vi "Single Video Display2.vi"() -> ()   [LabVIEW 2017]
uses:
  VideoWindowsCommand.ctl
panel:
  in  "Video Feed":enum16{"Camera 1", "Camera2", "Mobile"}(ring)=enum."Camera2"
  in  "MozillaBrowser 2":refnum<k7>(container)
  in  "Exit":bool
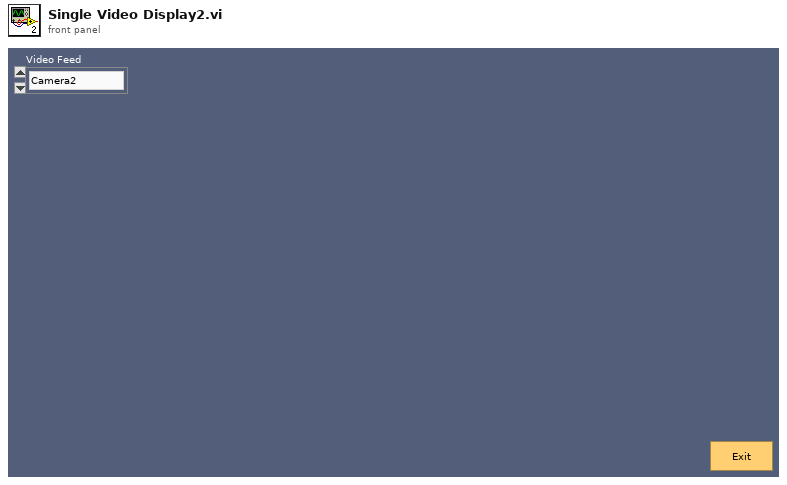
[diagram p1: front panel]
types:
  T1 = typedef "VideoWindowsCommand.ctl" = cluster{"Position":cluster{"Right":i32, "Bottom":i32}, "Exit":bool, "MoveToFront":bool}
  T2 = typedef "LVRectTypeDef.ctl" = cluster{"Left":i16, "Top":i16, "Right":i16, "Bottom":i16}
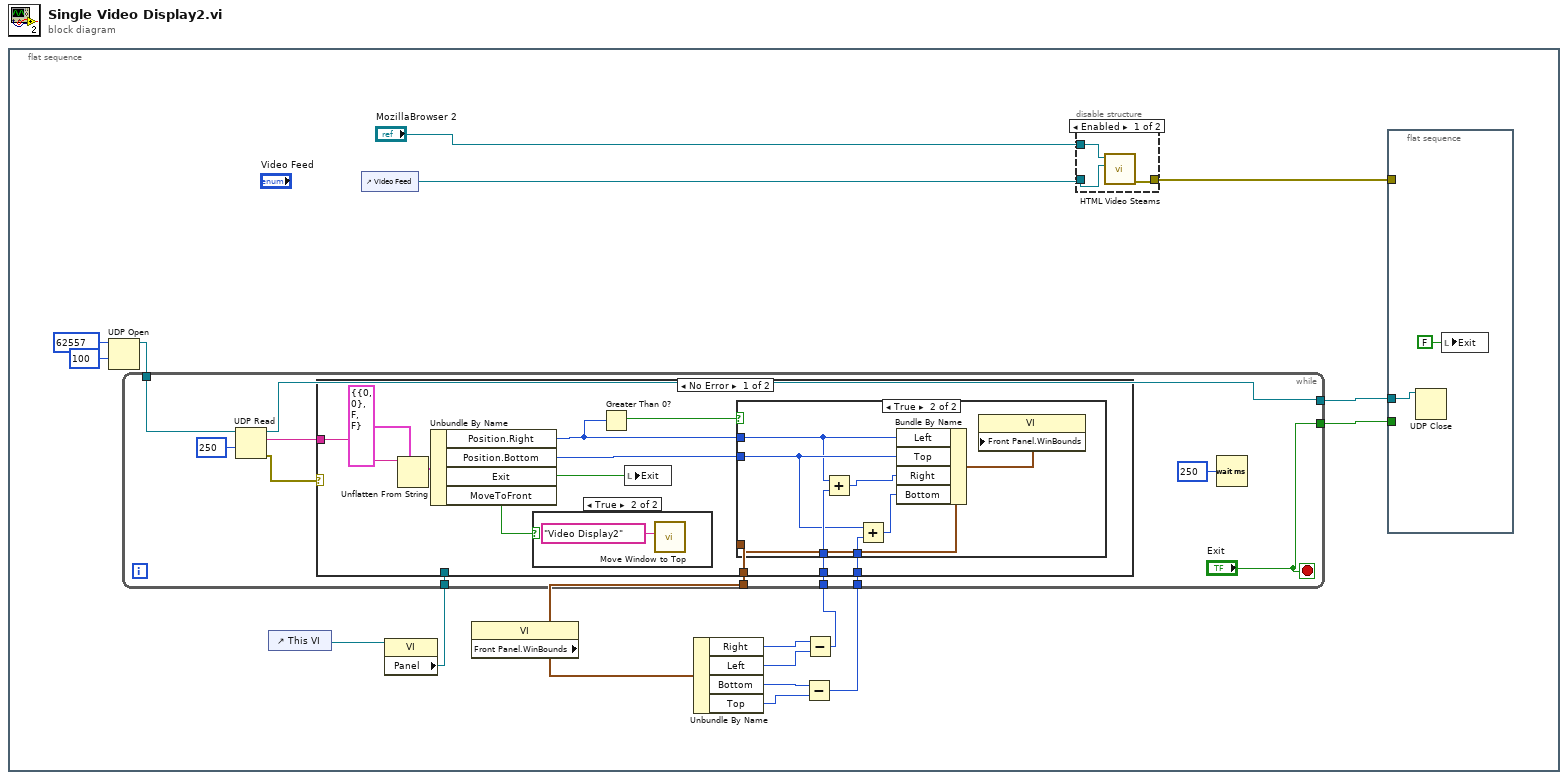
[diagram p0: block diagram]
diagram:
  n1 = flat-sequence {
    frame #0 {
      n2 = UDP Open(9:100 ("timeout ms (25000)"), 11:u16 62557 ("port")) -> (port=w12:refnum<k16>)  [unwired: 3 in, 2 out]
      n3 = control-ref of="This VI"() -> (w11:refnum<vi>)
      n4 = control-ref of="Video Feed"() -> (w16:refnum<vi>)
      n5 = property class="VI"(reference=w11) -> ("Panel"=w10:refnum<vi>)  [unwired: 1 in, 2 out]
      n6 = property class="VI"() -> ("Front Panel.WinBounds"=w3:T2)  [unwired: 2 in, 2 out]
      n7 = Unbundle By Name(w3) -> ("Right"=w6:i16, "Left"=w7:i16, "Bottom"=w4:i16, "Top"=w5:i16)
      n8 = Subtract(x=w4, y=w5) -> (x-y=w1:i16)
      n9 = Subtract(x=w6, y=w7) -> (x-y=w2:i16)
      n10 = while {
        tunnel: ["Exit"] -> w14
        tunnel: w12 -> [w28]
        tunnel: w10 -> [w24]
        tunnel: [w23] -> w9
        tunnel: w3 -> [w22]
        tunnel: w2 -> [w21]
        tunnel: w1 -> [w20]
        stop <- "Exit" stop-if-true
        n11 = UDP Read(connection ID=w28, timeout ms (25000)=250) -> (data out=w25:string, error out=w26:errorcluster, 3:w23:refnum<k16>)  [unwired: 2 in, 2 out]
        n12 = case shown="No Error" w26 {
          tunnel: w25 -> [w41 _]
          tunnel: w24 -> [_ _]
          tunnel: w22 -> [w37 _]
          tunnel: w21 -> [w36 _]
          tunnel: w20 -> [w34 _]
          frame No Error {
            n13 = Unflatten From String(type=T1 {"Position"={"Right"=0, "Bottom"=0}, "Exit"=FALSE, "MoveToFront"=FALSE}, binary string=w41) -> (value=w39:T1)  [unwired: 3 in, 2 out]
            n14 = Unbundle By Name(w39) -> ("Position.Right"=w33:i32, "Position.Bottom"=w35:i32, "Exit"=w38:bool, "MoveToFront"=w31:bool)
            n15 = case shown="True" w31 {
              frame False {
              }
              frame True {
                n16 = call "Move Window to Top.vi"("window name (\"\")"="Video Display2" ("window name (\"\")")) -> ()  [unwired: 5 in, 2 out]
              }
            }
            n17 = Greater Than 0?(x=w33) -> (x > 0?=w32:bool)
            n18 = local write "Exit"(w38) -> ()
            n19 = case shown="True" w32 {
              tunnel: w37 -> [_ w50]
              tunnel: w36 -> [_ w49]
              tunnel: w35 -> [_ w47]
              tunnel: w34 -> [_ w46]
              tunnel: w33 -> [_ w43]
              frame False {
              }
              frame True {
                n20 = Add(x=w43, y=w49) -> (x+y=w48:i32)
                n21 = Add(x=w47, y=w46) -> (x+y=w45:i32)
                n22 = Bundle By Name(cluster=w50, "Left"=w43, "Top"=w47, "Right"=w48, "Bottom"=w45) -> (w44:T2)
                n23 = property class="VI"("Front Panel.WinBounds"=w44) -> ()  [unwired: 2 in, 2 out]
              }
            }
          }
          frame Error {
          }
        }
        n24 = Wait (ms)(milliseconds to wait=u32 250) -> ()  [unwired: 1 out]
      }
      n25 = disable-structure shown="Enabled" {
        disable-tunnel: "MozillaBrowser 2" -> [w53 _]
        disable-tunnel: w16 -> [w52 _]
        disable-tunnel: [w51 _] -> w15
        frame Enabled {
          n26 = call "HTML Video Steams.vi"("Video Feed 2"=w52, "Automation Refnum in"=w53) -> ("error out"=w51:errorcluster)  [unwired: 8 in, 1 out]
        }
        frame Disabled {
        }
      }
      n27 = flat-sequence {
        tunnel: w15 -> [_]
        tunnel: w14 -> [_]
        tunnel: w9 -> [w18]
        frame #0 {
          n28 = UDP Close(connection ID=w18) -> ()  [unwired: 1 in, 2 out]
          n29 = local write "Exit"(FALSE ("Exit")) -> ()
        }
      }
    }
  }
